vi "Unbundle and Calc Fresnel.vi"(8 "error in (no error)":errorcluster, 9 "SLM Params":T2 {"Centre X" format="%.3g"; "Centre Y" format="%.3g"}, 10 "Spot Settings":T1, 11 "holo_init":u8[](array[numeric])) -> (0 "error out":errorcluster, 3 "Fresnel holo":u8[](array[numeric]))   [LabVIEW 2020]
uses:
  _controls/PCIe SLM params.ctl
  <userlib>/SLM ImageGen/SLM ImageGen.lvlib
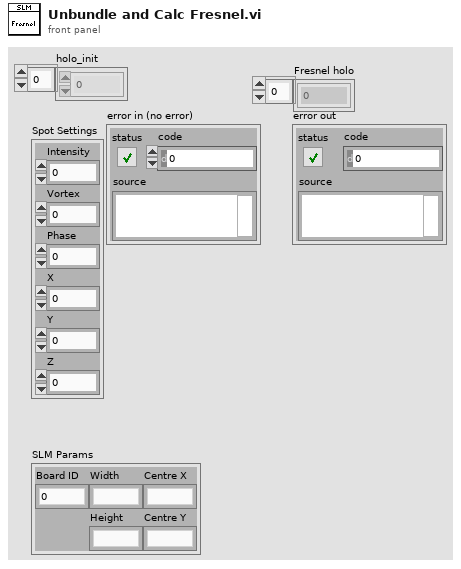
[diagram p1: front panel]
types:
  T1 = cluster{"Intensity":dbl, "Vortex":dbl, "Phase":dbl, "X":dbl, "Y":dbl, "Z":dbl}
  T2 = typedef "PCIe SLM params.ctl" = cluster{"Width":dbl, "Height":dbl, "Board ID":i32, "Centre Y":dbl, "Centre X":dbl}
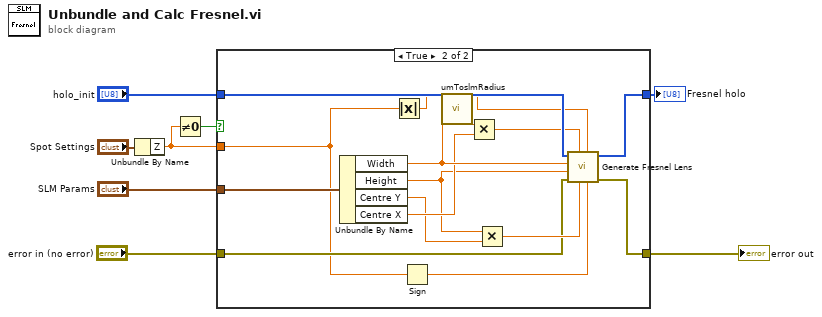
[diagram p0: block diagram]
diagram:
  n1 = Unbundle By Name("Spot Settings") -> ("Z"=w7:dbl)
  n2 = Not Equal To 0?(x=w7) -> (x != 0?=w5:bool)
  n3 = case shown="True" w5 {
    tunnel: "holo_init" -> [w10 w24]
    tunnel: [w10 w23] -> w4
    tunnel: w7 -> [_ w12]
    tunnel: "SLM Params" -> [_ w22]
    tunnel: [w9 w15] -> w2
    tunnel: "error in (no error)" -> [w9 w14]
    frame False {
    }
    frame True {
      n4 = Unbundle By Name(w22) -> ("Width"=w21:dbl, "Height"=w18:dbl, "Centre Y"=w17:dbl, "Centre X"=w20:dbl)
      n5 = Absolute Value(x=w12) -> (abs(x)=w11:dbl)
      n6 = Sign(1:w12) -> (0:w13:dbl)
      n7 = call "umToslmRadius.vi"() -> ()  [unwired: 1 in, 1 out]
      n8 = Multiply(x=w21, y=w20) -> (x*y=w19:dbl)
      n9 = Multiply(x=w18, y=w17) -> (x*y=w16:dbl)
      n10 = call <userlib>:"Generate Fresnel Lens.vi"("Power"=w13, "radius"=w11, "centerY"=w16, "centerX"=w19, "error in (no error)"=w14, "height"=w18, "width"=w21, "Array"=w24) -> ("error out"=w15:errorcluster, "Array out"=w23:u8[])  [unwired: 2 in]
    }
  }
  "Fresnel holo" <- w4
  "error out" <- w2
